vi "Test.vi"() -> ()   [LabVIEW 2014]
panel:
  out "Numeric":i32
  in  "stop":bool
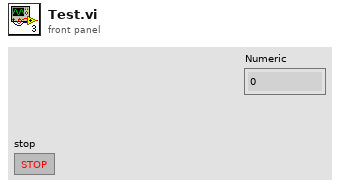
[diagram p1: front panel]
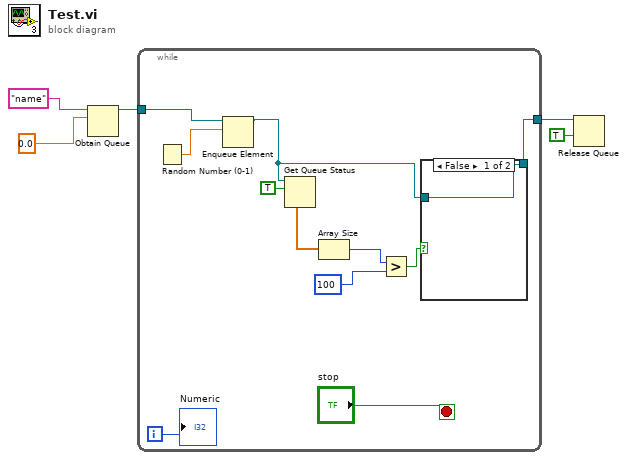
[diagram p0: block diagram]
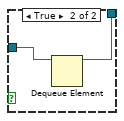
[diagram p2: hidden frame]
diagram:
  n1 = Obtain Queue(name (unnamed)="name", element data type=0.0) -> (queue out=w5:refnum<queue>)  [unwired: 3 in, 2 out]
  n2 = while {
    tunnel: w5 -> [w16]
    tunnel: [w7] -> w1
    i -> [w6]
    stop <- "stop" stop-if-true
    n3 = Random Number (0-1)() -> (number: 0 to 1=w15:dbl)
    n4 = Enqueue Element(queue=w16, element=w15) -> (queue out=w8:refnum<queue>)  [unwired: 2 in, 2 out]
    n5 = Get Queue Status(queue=w8, return elements? (F)=TRUE) -> (elements=w12:dbl[])  [unwired: 1 in, 7 out]
    n6 = Array Size(array=w12) -> (size(s)=w11:i32)
    n7 = Greater?(x=w11, y=100) -> (0:w9:bool)
    n8 = case shown="False" w9 {
      tunnel: w8 -> [w17 w19]
      tunnel: [w17 w18] -> w7
      frame False {
      }
      frame True {
        n9 = Dequeue Element(queue=w19) -> (queue out=w18:refnum<queue>)  [unwired: 2 in, 3 out]
      }
    }
    "Numeric" <- w6
  }
  n10 = Release Queue(queue=w1, force destroy? (F)=TRUE) -> ()  [unwired: 1 in, 3 out]
